vi "Create JKI REST Client.vi"(4 "Default Headers ([JSON])":T1[](array[typedef])=[{"header"="Content-Type", "value"="application/json"}], 5 "REST Client in":refnum<class "REST Client_JKI.lvclass">, 6 "Verify Server(true)":bool=TRUE, 7 "Cookie File":path, 8 "error in (no error)":errorcluster, 9 "Authentication":cluster{"Username":string, "Password":string}, 10 "Escape URLs (true)":bool=TRUE, 11 "Base URL":string) -> (0 "error out":errorcluster, 3 "REST Client out":refnum<class "REST Client_JKI.lvclass">)   [LabVIEW 2018, in "REST Client.lvlib" / "REST Client_JKI.lvclass"]
doc: "The VI provides multiple arguments for defining how to create the JKI REST Client instance.\n\n<b>Base URL</b> specifies the base URL to be used for the HTTP requests.\n\n<b>Escape URLs</b> when true instruct the REST Client to escape all URLs before executing the requests. If you have already escaped the URLs, set this to false.\n\n<b>Authentication</b> allows setting the username and password for services that use HTTP authentication.\n\n<b>Verify Server</b> when true instructs the REST Client to validate the certificate of the server when HTTPS protocol is being used.\n\n<b>Default Headers</b> specifies an array of headers to be used with every requests. Defaults to application/json content type.\n\n<b>Cookie File</b> specifies a file path to be used for cookies."
uses:
  REST Client_JKI.lvclass
  C:/Viviota/Projects/R&D/LabVIEW_HTTP_REST_Client/source/classes/REST Client/REST Client.lvclass
  REST Client/HTTP Header.ctl
  REST Client_JKI.lvclass/REST Client_JKI.ctl
  REST Client/REST Client.lvclass
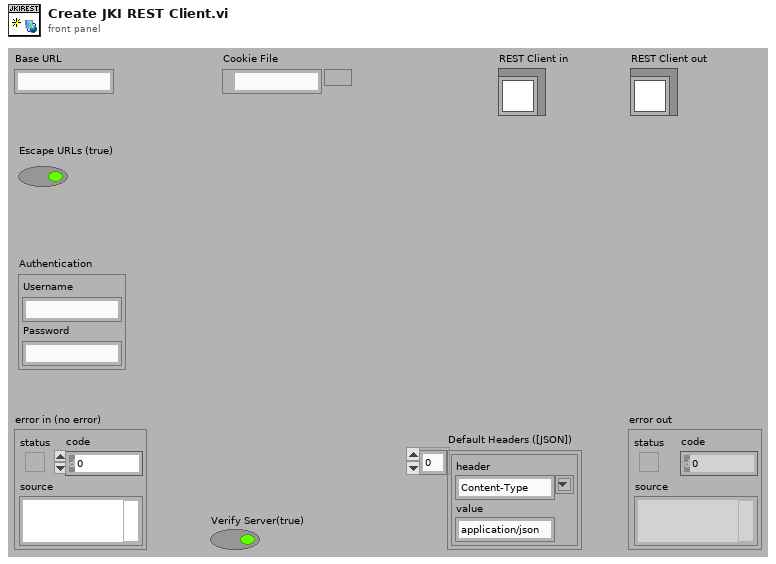
[diagram p1: front panel]
types:
  T1 = typedef "REST Client.lvlib/REST Client.lvclass/HTTP Header.ctl" = cluster{"header":string, "value":string}
  T2 = typedef "LabVIEWHTTPClient.lvlib/ClientHandle.ctl" = refnum<k1>
  T3 = cluster{"client handle out":T2, "Default Headers ([JSON])":T1[]}
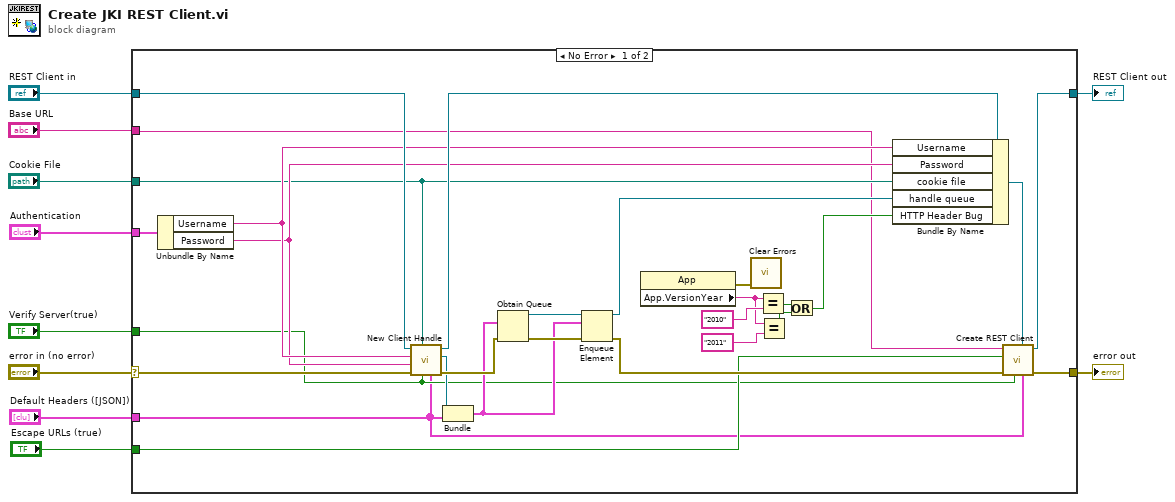
[diagram p0: block diagram]
diagram:
  n1 = case shown="No Error" "error in (no error)" {
    selector: "error in (no error)" -> [w38 w40]
    tunnel: [w18 w40] -> w9
    tunnel: [w17 w39] -> w7
    tunnel: "REST Client in" -> [w37 w39]
    tunnel: "Cookie File" -> [w15 _]
    tunnel: "Verify Server(true)" -> [w12 _]
    tunnel: "Default Headers ([JSON])" -> [w11 _]
    tunnel: "Authentication" -> [w22 _]
    tunnel: "Base URL" -> [w14 _]
    tunnel: "Escape URLs (true)" -> [w13 _]
    frame No Error {
      n2 = Unbundle By Name(w22) -> ("Username"=w21:string, "Password"=w20:string)
      n3 = call "New Client Handle.vi"("headers"=w11, "verify server(true)"=w12, "cookie file"=w15, "error in (no error)"=w38, "password"=w20, "username"=w21, "REST Client in"=w37) -> ("error out"=w35:errorcluster, "client handle out"=w32:T2, "REST Client out"=w36:refnum<class "REST Client_JKI.lvclass">)  [unwired: 2 in]
      n4 = Bundle("client handle out"=w32, "Default Headers ([JSON])"=w11) -> (w31:T3)  [unwired: 1 in]
      n5 = Obtain Queue(element data type=w31, error in (no error)=w35) -> (queue out=w34:refnum<queue>, error out=w33:errorcluster)  [unwired: 3 in, 1 out]
      n6 = Enqueue Element(queue=w34, element=w31, error in (no error)=w33) -> (queue out=w30:refnum<queue>, error out=w19:errorcluster)  [unwired: 1 in, 1 out]
      n7 = property class="App"() -> (error out=w23:errorcluster, "App.VersionYear"=w26:string)  [unwired: 2 in, 1 out]
      n8 = call <vilib>:"Clear Errors.vi"("error in (no error)"=w23) -> ()  [unwired: 5 in, 2 out]
      n9 = Equal?(x=w26, y="2010") -> (x = y?=w28:bool)
      n10 = Equal?(x=w26, y="2011") -> (x = y?=w27:bool)
      n11 = Or(x=w28, y=w27) -> (x .or. y?=w24:bool)
      n12 = Bundle By Name(cluster=w36, "Username"=w21, "Password"=w20, "cookie file"=w15, "handle queue"=w30, "HTTP Header Bug"=w24) -> (w16:refnum<class "REST Client_JKI.lvclass">)
      n13 = call "Create REST Client.vi"("Default Headers ([JSON])"=w11, "REST Client in"=w16, "Verify Server(true)"=w12, "error in (no error)"=w19, "Escape URLs (true)"=w13, "Base URL"=w14) -> ("error out"=w18:errorcluster, "REST Client out"=w17:refnum<class "REST Client_JKI.lvclass">)  [unwired: 4 in]
    }
    frame Error {
    }
  }
  "error out" <- w9
  "REST Client out" <- w7
